vi "POP_Make Popup Visible.vi"(6 "LV Version":string, 7 "Popup Parameters":T1={"Prop Type"=enum."Unkown", "Initial Value"=variant, "Caption Strings"=[], "Ring Strings"=[], "Cell Rect"={"left"=0, "top"=0, "right"=0, "bottom"=0}, "Mouse Coords"={"x"=0, "y"=0}, "Call Data"=variant, "Ring Values"=[], "Browse Options"={"Prompt"="", "Match Pattern"="", "Mode"=enum."existing file", "Start Path"=path "", "Pattern Label"="", "Button Text"=""}, "Combo Box"={"Allow Undefined Strings"=FALSE}}, 8 "error in (no error)":errorcluster, 9 "Ctl Offsets":cluster{"Left":i32, "Top":i32}[](array[cluster]), 11 "Popup Cluster Ref":refnum<vi>) -> (0 "error out":errorcluster, 2 "event data":T4)   [LabVIEW 2016]
uses:
  Ctrls/POP_Monitor Register Data.ctl
  Ctrls/POP_Event Enum.ctl
  Ctrls/POP_Popup Call Parameters.ctl
  Ctrls/POP_Data Type.ctl
  <vilib>/Utility/miscctls.llb/LVBrowseOptionsTypeDef.ctl
  <vilib>/Utility/miscctls.llb/LVStringsAndValuesArrayTypeDef.ctl
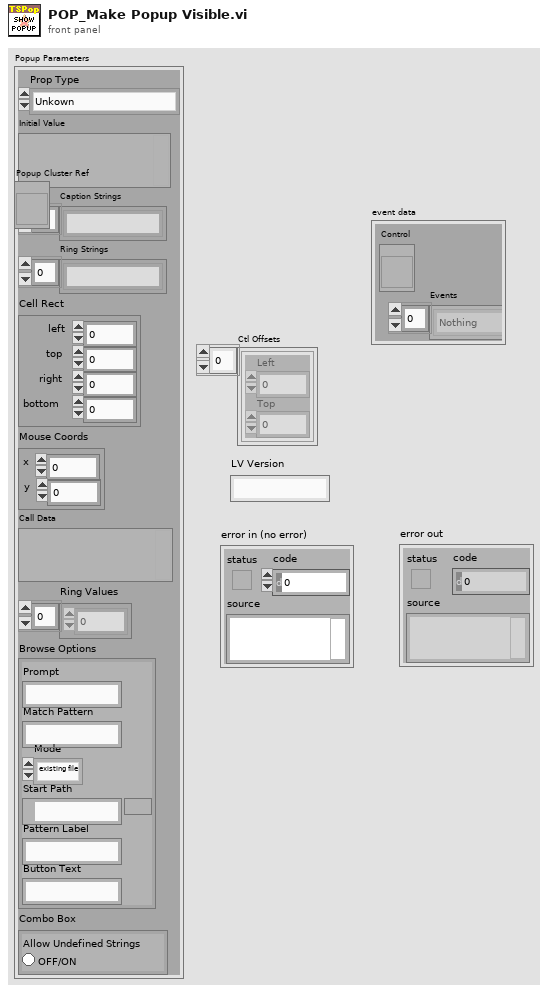
[diagram p1: front panel]
types:
  T1 = typedef "POP_Popup Call Parameters.ctl" = cluster{"Prop Type":T2, "Initial Value":variant, "Caption Strings":string[], "Ring Strings":string[], "Cell Rect":cluster{"left":i16, "top":i16, "right":i16, "bottom":i16}, "Mouse Coords":cluster{"x":i16, "y":i16}, "Call Data":variant, "Ring Values":ext[], "Browse Options":T3, "Combo Box":cluster{"Allow Undefined Strings":bool}}
  T2 = typedef "POP_Data Type.ctl" = enum16{"NO POPUP", "Unkown", "String", "Integer", "Float", "Color", "Boolean", "Ring", "Captioned String", "Captioned Integer", "Button Color", "2 Int Cluster", "4 Int Cluster", "6-Dbl Cluster", "Path", "Combox", "Time", "ShotCut String"}
  T3 = typedef "LVBrowseOptionsTypeDef.ctl" = cluster{"Prompt":string, "Match Pattern":string, "Mode":enum32{"existing file", "new file", "new or existing file", "existing dir", "new dir", "new or existing dir", "existing file (use LLBs)", "new file (use LLBs)", "new or existing file (use LLBs)", "new or existing file or directory (use LLBs)", "existing dir (use LLBs)", "new dir (use LLBs)", "new or existing dir (use LLBs)", "existing file or dir", "new file or dir", "new or existing file or dir", "existing file or dir (use LLBs)", "new file or dir (use LLBs)"}, "Start Path":path, "Pattern Label":string, "Button Text":string}
  T4 = typedef "POP_Monitor Register Data.ctl" = cluster{"Control":refnum<vi>, "Events":T5[]}
  T5 = typedef "POP_Event Enum.ctl" = enum16{"Nothing", "Enter Key Accept", "Escape Key Cancel", "Mouse Outside Accept", "Mouse Outside Cancel", "Mouse Move Accept", "Mouse Move Cancel", "Mouse Leave Cancel", "Value Change Accept", "Lose Focus Cancel", "Cancel Button", "Accept Button", "Shift Ctrl Key Down"}
  T6 = typedef "LVStringsAndValuesArrayTypeDef.ctl" = cluster{"String":string, "Value":ext}[]
  T7 = cluster{"left":i32, "top":i32, "right":i32, "bottom":i32}
  T8 = cluster{"a0":dbl, "a1":dbl, "a2":dbl, "a3":dbl, "a4":dbl, "a5":dbl}
  T9 = cluster{"left":i16, "top":i16, "right":i16, "bottom":i16}
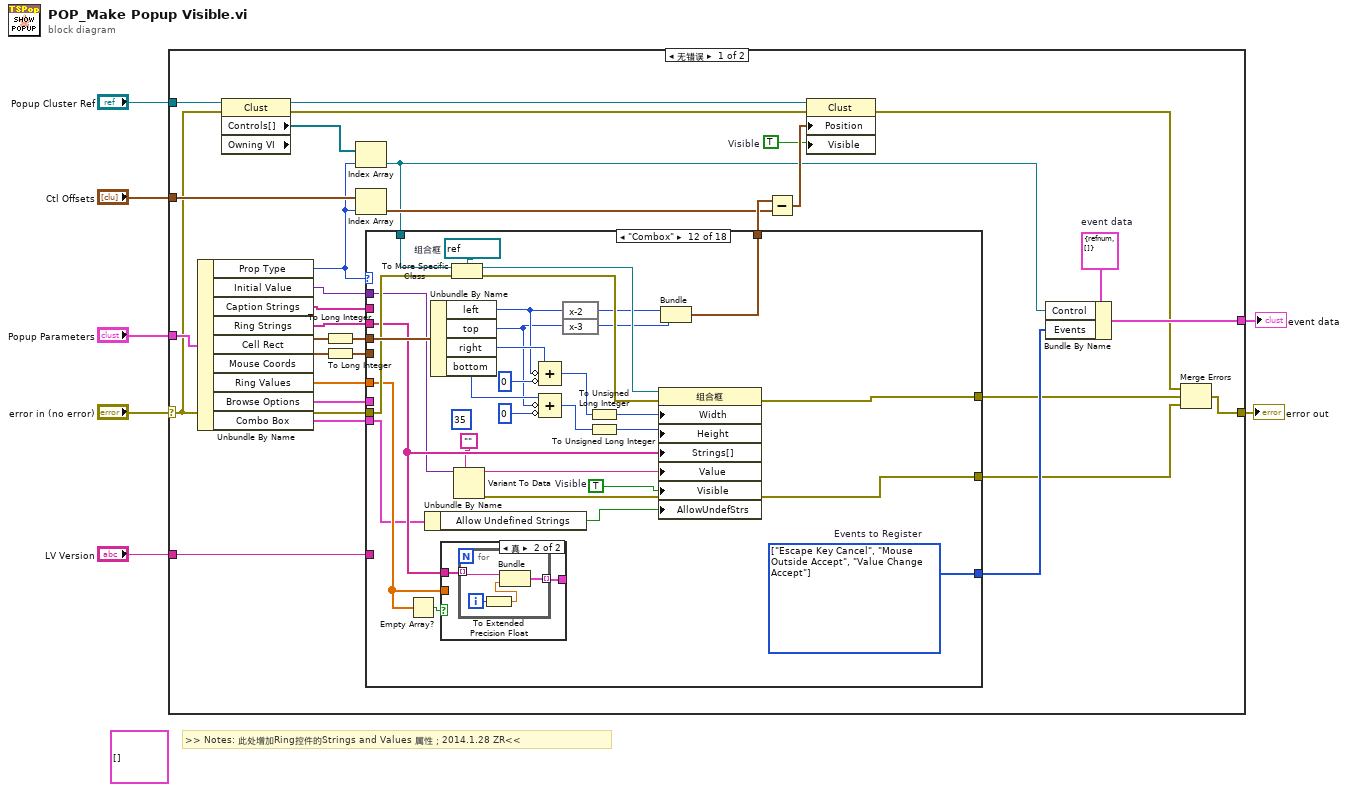
[diagram p0: block diagram]
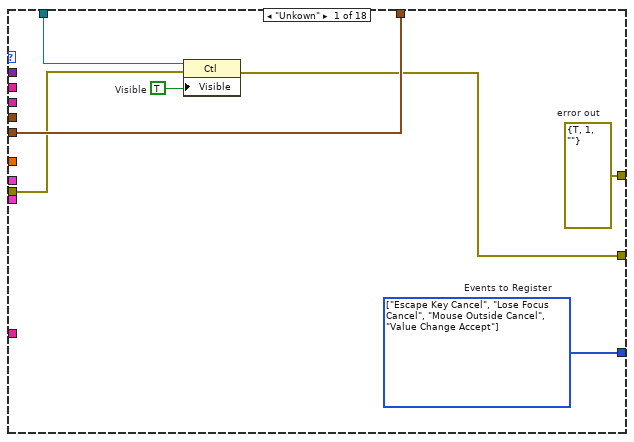
[diagram p2: hidden frame]
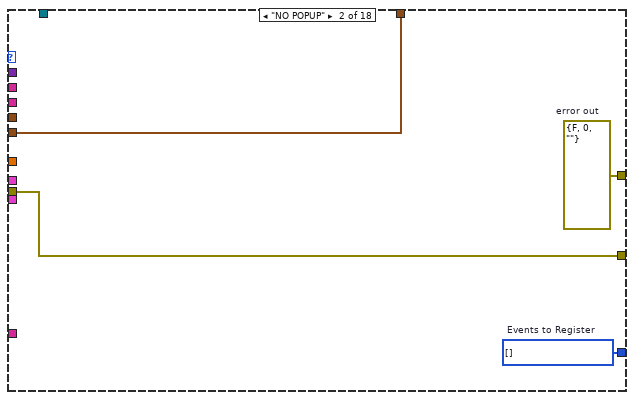
[diagram p3: hidden frame]
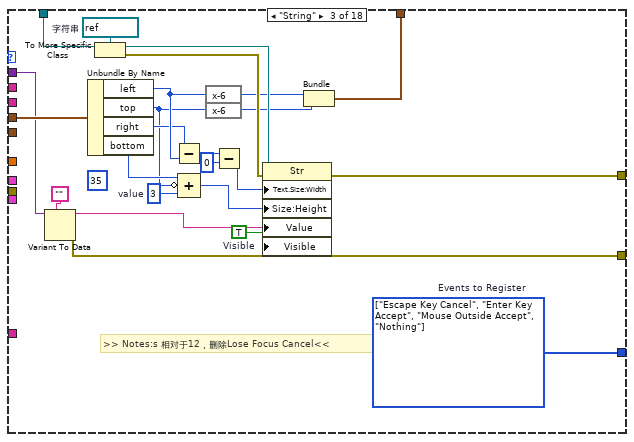
[diagram p4: hidden frame]
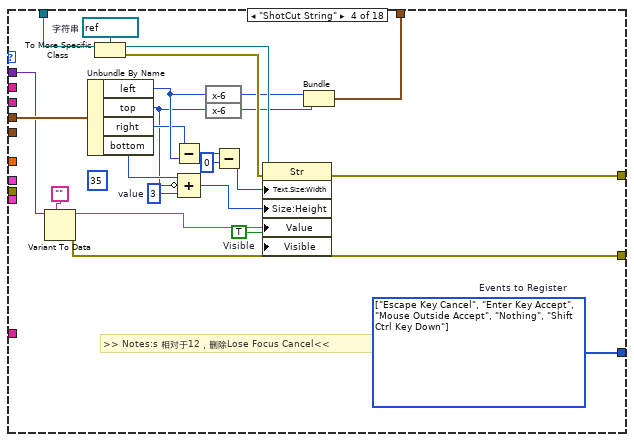
[diagram p5: hidden frame]
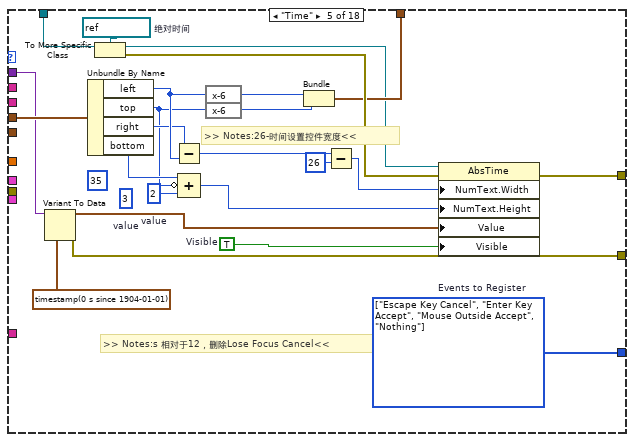
[diagram p6: hidden frame]
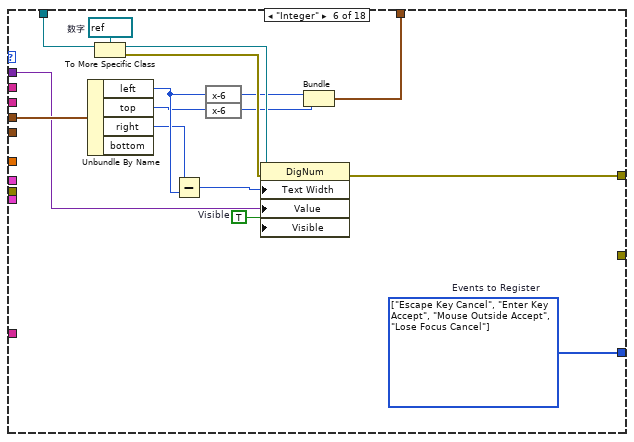
[diagram p7: hidden frame]
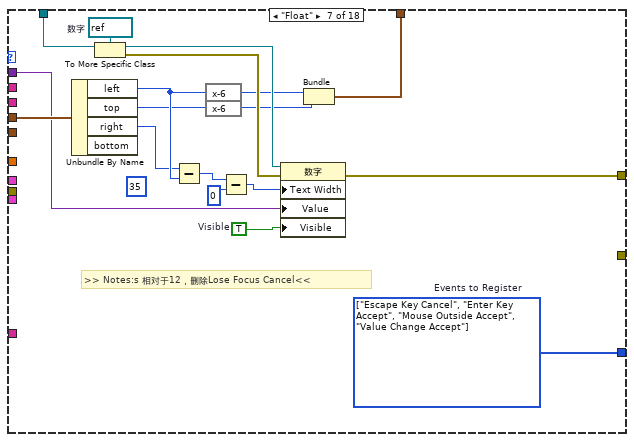
[diagram p8: hidden frame]
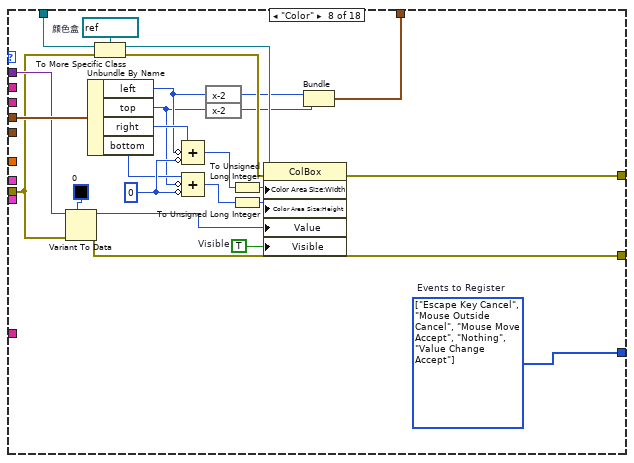
[diagram p9: hidden frame]
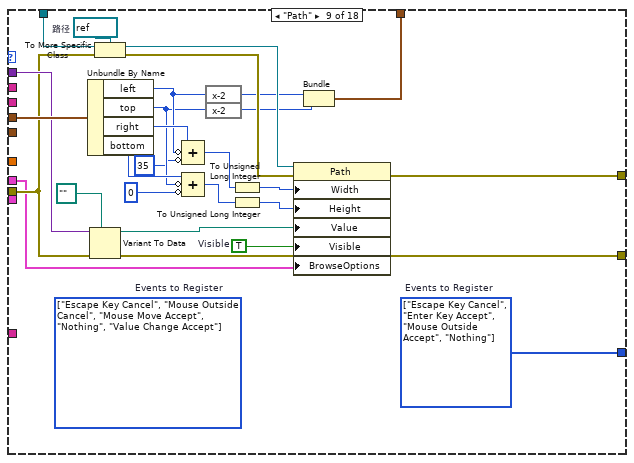
[diagram p10: hidden frame]
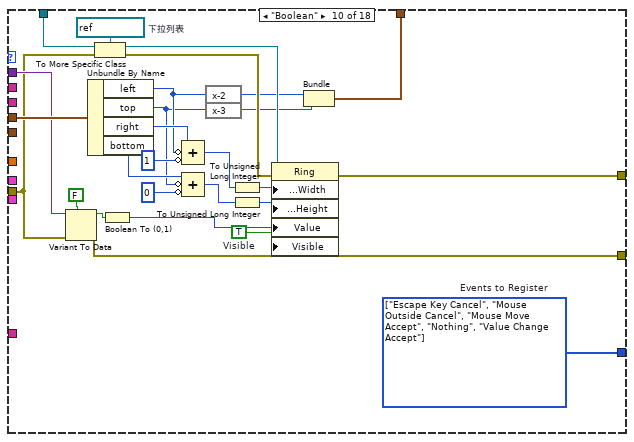
[diagram p11: hidden frame]
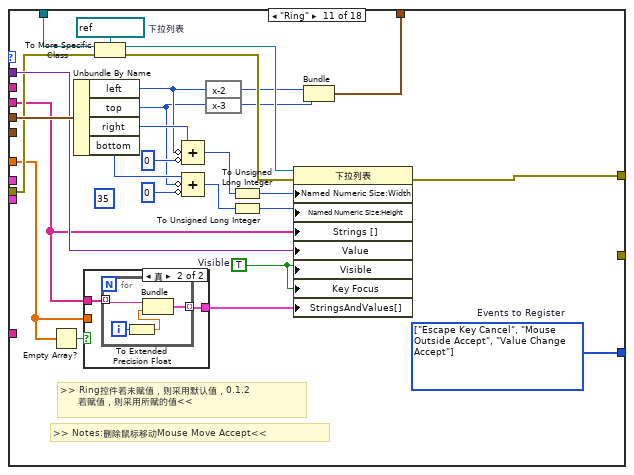
[diagram p12: hidden frame]
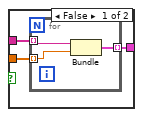
[diagram p13: hidden frame]
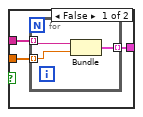
[diagram p14: hidden frame]
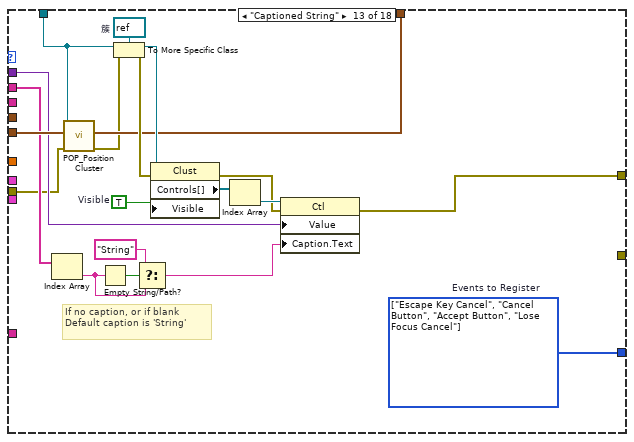
[diagram p15: hidden frame]
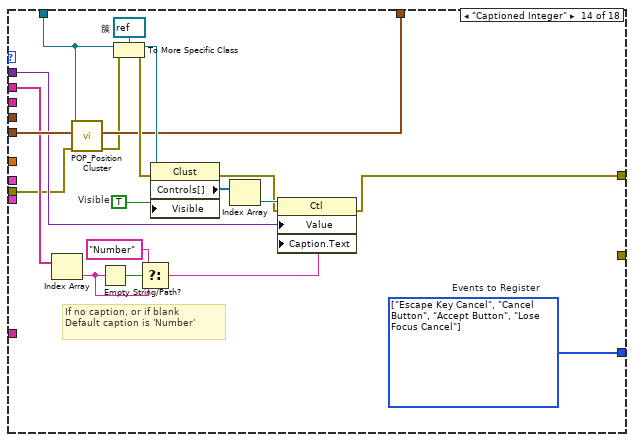
[diagram p16: hidden frame]
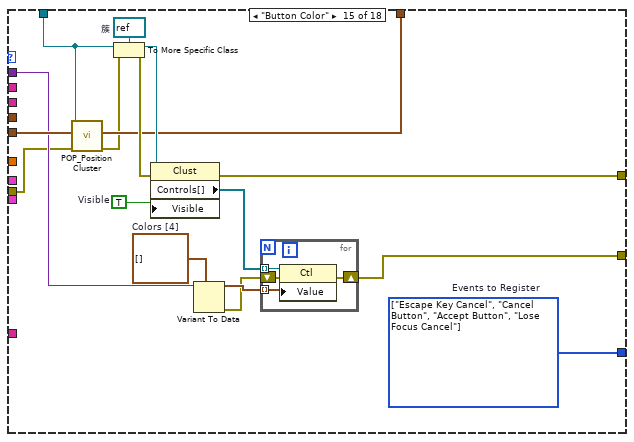
[diagram p17: hidden frame]
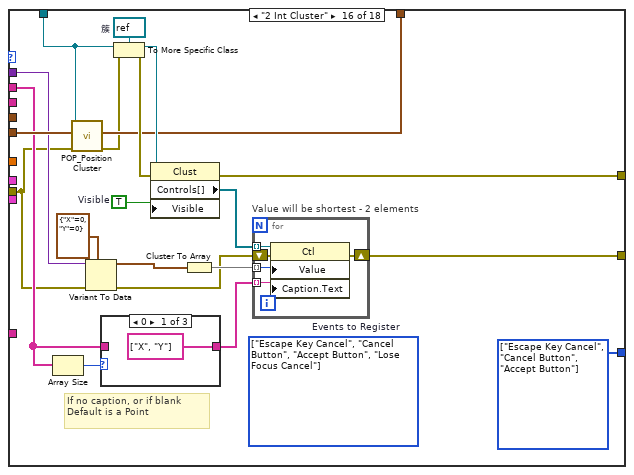
[diagram p18: hidden frame]
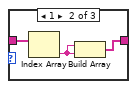
[diagram p19: hidden frame]
diagram:
  (unwired) T6 [] ("Strings And Values []")
  # ">> Notes: 此处增加Ring控件的Strings and Values 属性；2014.1.28 ZR<<"
  n1 = case shown="无错误" "error in (no error)" {
    selector: "error in (no error)" -> [w12 w490]
    tunnel: "Popup Parameters" -> [w38 _]
    tunnel: "Popup Cluster Ref" -> [w37 _]
    tunnel: "Ctl Offsets" -> [w35 _]
    tunnel: [w24 w489] -> w4
    tunnel: [w17 w490] -> w2
    tunnel: "LV Version" -> [w13 _]
    frame No Error {
      w34 = T4 {"Control"=refnum, "Events"=[]}  # event data
      w11 = TRUE  # Visible
      n2 = Unbundle By Name(w38) -> ("Prop Type"=w32:T2, "Initial Value"=w33:variant, "Caption Strings"=w22:string[], "Ring Strings"=w23:string[], "Cell Rect"=w30:T9, "Mouse Coords"=w15:cluster{"x":i16, "y":i16}, "Ring Values"=w10:ext[], "Browse Options"=w9:T3, "Combo Box"=w8:cluster{"Allow Undefined Strings":bool})
      n3 = property class="Clust" props=["Controls[]", "Owning VI"](reference=w37, error in=w12) -> (reference out=w31:refnum<vi>, error out=w21:errorcluster, "Controls[]"=w36:refnum<vi>[])  [unwired: 1 out]
      n4 = To Long Integer(number=w30) -> (32bit integer=w16:T7)
      n5 = To Long Integer(number=w15) -> (32bit integer=w14:cluster{"x":i32, "y":i32})
      n6 = Index Array(array=w36, index=w32) -> (element=w25:refnum<vi>)
      n7 = Index Array(array=w35, index=w32) -> (element=w28:cluster{"Left":i32, "Top":i32})
      n8 = case shown="\"Combox\"" w32 {
        tunnel: w25 -> [w42 _ w63 w87 w112 w133 w153 w179 w206 w232 w260 w303 w326 w346 w365 w391 w421 w461]
        tunnel: w33 -> [_ _ w66 w90 w114 w123 w143 w170 w198 w224 w242 w278 w327 w347 w362 w390 w420 w460]
        tunnel: w16 -> [_ _ w67 w91 w115 w134 w154 w180 w207 w233 w261 w304 _ _ _ _ _ _]
        tunnel: [w45 w49 w59 w83 w109 w129 w149 w175 w202 w228 w256 w299 w319 w338 w370 w395 w426 w466] -> w19
        tunnel: [w44 w47 w56 w80 w106 w126 w146 w172 w199 w225 w253 w296 w330 w350 w366 w392 w422 w462] -> w29
        tunnel: [w43 w48 w55 w79 w105 w125 w145 w158 w183 w209 w240 w284 w333 w353 w369 w378 w425 w465] -> w26
        tunnel: w23 -> [_ _ _ _ _ _ _ _ _ _ w238 w282 _ _ _ _ _ _]
        tunnel: w14 -> [w44 w47 _ _ _ _ _ _ _ _ _ _ w331 w351 w367 w393 w423 w463]
        tunnel: w22 -> [_ _ _ _ _ _ _ _ _ _ _ _ w325 w345 _ w388 w418 w458]
        tunnel: [w39 w46 w52 w76 w102 _ _ w159 w188 w210 _ w276 _ _ w358 w384 w410 w451] -> w18
        tunnel: w13 -> [_ _ _ _ _ _ _ _ _ _ _ _ _ _ _ _ _ _]
        tunnel: w12 -> [w40 w46 _ _ _ _ _ w157 w187 w208 w241 w285 w317 w337 w357 w379 w409 w450]
        tunnel: w10 -> [_ _ _ _ _ _ _ _ _ _ w236 w281 _ _ _ _ _ _]
        tunnel: w9 -> [_ _ _ _ _ _ _ _ w181 _ _ _ _ _ _ _ _ _]
        tunnel: w8 -> [_ _ _ _ _ _ _ _ _ _ _ w275 _ _ _ _ _ _]
        frame "Unkown" {
          w43 = T5[] [enum."Escape Key Cancel", enum."Lose Focus Cancel", enum."Mouse Outside Cancel", enum."Value Change Accept"] items=["Nothing", "Enter Key Accept", "Escape Key Cancel", "Mouse Outside Accept", "Mouse Outside Cancel", "Mouse Move Accept", "Mouse Move Cancel", "Mouse Leave Cancel", "Value Change Accept", "Lose Focus Cancel", "Cancel Button", "Accept Button", "Shift Ctrl Key Down"]  # Events to Register
          w45 = errorcluster {"status"=TRUE, "code"=1, "source"=""}  # error out
          w41 = TRUE  # Visible
          n9 = property class="Ctl"(reference=w42, error in=w40, "Visible"=w41) -> (error out=w39:errorcluster)  [unwired: 1 out]
        }
        frame "NO POPUP" {
          w48 = T5[] [] items=["Nothing", "Enter Key Accept", "Escape Key Cancel", "Mouse Outside Accept", "Mouse Outside Cancel", "Mouse Move Accept", "Mouse Move Cancel", "Mouse Leave Cancel", "Value Change Accept", "Lose Focus Cancel", "Cancel Button", "Accept Button", "Shift Ctrl Key Down"]  # Events to Register
          w49 = errorcluster {"status"=FALSE, "code"=0, "source"=""}  # error out
        }
        frame "String" {
          (unwired) 35 ("y")
          w62 = refnum<vi> refnum  # 字符串
          w68 = TRUE  # Visible
          w69 = 3  # value
          w55 = T5[] [enum."Escape Key Cancel", enum."Enter Key Accept", enum."Mouse Outside Accept", enum."Nothing"] items=["Nothing", "Enter Key Accept", "Escape Key Cancel", "Mouse Outside Accept", "Mouse Outside Cancel", "Mouse Move Accept", "Mouse Move Cancel", "Mouse Leave Cancel", "Value Change Accept", "Lose Focus Cancel", "Cancel Button", "Accept Button", "Shift Ctrl Key Down"]  # Events to Register
          # ">> Notes:s 相对于12，删除Lose Focus Cancel<<"
          n10 = Variant To Data(type="", Variant=w66) -> (data=w64:string, error out=w52:errorcluster)  [unwired: 1 in]
          n11 = Unbundle By Name(w67) -> ("left"=w71:i32, "top"=w53:i32, "right"=w54:i32, "bottom"=w73:i32)
          n12 = To More Specific Class(target class=w62, reference=w63) -> (specific class reference=w61:refnum<vi>, error out=w60:errorcluster)  [unwired: 1 in]
          n13 = Subtract(x=w54, y=w71) -> (x-y=w70:i32)
          n14 = Compound Arithmetic op=ADD(w73, invert w53, w69) -> (w72:i32)
          n15 = expression code="x-6"(w71) -> (w58:i32)
          n16 = expression code="x-6"(w53) -> (w57:i32)
          n17 = Subtract(x=w70, y=0) -> (x-y=w51:i32)
          n18 = property class="Str"(reference=w61, error in=w60, "Text.Size:Width"=w51, "Size:Height"=w72, "Value"=w64, "Visible"=w68) -> (error out=w59:errorcluster)  [unwired: 1 out]
          n19 = Bundle("left"=w58, "top"=w57) -> (w56:cluster{"left":i32, "top":i32})  [unwired: 1 in]
        }
        frame "ShotCut String" {
          (unwired) 35 ("y")
          w86 = refnum<vi> refnum  # 字符串
          w92 = TRUE  # Visible
          w93 = 3  # value
          w79 = T5[] [enum."Escape Key Cancel", enum."Enter Key Accept", enum."Mouse Outside Accept", enum."Nothing", enum."Shift Ctrl Key Down"] items=["Nothing", "Enter Key Accept", "Escape Key Cancel", "Mouse Outside Accept", "Mouse Outside Cancel", "Mouse Move Accept", "Mouse Move Cancel", "Mouse Leave Cancel", "Value Change Accept", "Lose Focus Cancel", "Cancel Button", "Accept Button", "Shift Ctrl Key Down"]  # Events to Register
          # ">> Notes:s 相对于12，删除Lose Focus Cancel<<"
          n20 = Variant To Data(type="", Variant=w90) -> (data=w88:string, error out=w76:errorcluster)  [unwired: 1 in]
          n21 = Unbundle By Name(w91) -> ("left"=w95:i32, "top"=w77:i32, "right"=w78:i32, "bottom"=w97:i32)
          n22 = To More Specific Class(target class=w86, reference=w87) -> (specific class reference=w85:refnum<vi>, error out=w84:errorcluster)  [unwired: 1 in]
          n23 = Subtract(x=w78, y=w95) -> (x-y=w94:i32)
          n24 = Compound Arithmetic op=ADD(w97, invert w77, w93) -> (w96:i32)
          n25 = expression code="x-6"(w95) -> (w82:i32)
          n26 = expression code="x-6"(w77) -> (w81:i32)
          n27 = Subtract(x=w94, y=0) -> (x-y=w75:i32)
          n28 = property class="Str"(reference=w85, error in=w84, "Text.Size:Width"=w75, "Size:Height"=w96, "Value"=w88, "Visible"=w92) -> (error out=w83:errorcluster)  [unwired: 1 out]
          n29 = Bundle("left"=w82, "top"=w81) -> (w80:cluster{"left":i32, "top":i32})  [unwired: 1 in]
        }
        frame "Time" {
          (unwired) 3  # value
          (unwired) 35 ("y")
          w111 = refnum<vi> refnum  # 绝对时间
          w116 = TRUE  # Visible
          w117 = 2  # value
          w105 = T5[] [enum."Escape Key Cancel", enum."Enter Key Accept", enum."Mouse Outside Accept", enum."Nothing"] items=["Nothing", "Enter Key Accept", "Escape Key Cancel", "Mouse Outside Accept", "Mouse Outside Cancel", "Mouse Move Accept", "Mouse Move Cancel", "Mouse Leave Cancel", "Value Change Accept", "Lose Focus Cancel", "Cancel Button", "Accept Button", "Shift Ctrl Key Down"]  # Events to Register
          # ">> Notes:26-时间设置控件宽度<<"
          # ">> Notes:s 相对于12，删除Lose Focus Cancel<<"
          n30 = Variant To Data(type=timestamp(0 s since 1904-01-01) ("Time"), Variant=w114) -> (data=w113:timestamp, error out=w102:errorcluster)  [unwired: 1 in]
          n31 = Unbundle By Name(w115) -> ("left"=w119:i32, "top"=w103:i32, "right"=w104:i32, "bottom"=w121:i32)
          n32 = To More Specific Class(target class=w111, reference=w112) -> (specific class reference=w98:refnum<vi>, error out=w110:errorcluster)  [unwired: 1 in]
          n33 = Subtract(x=w104, y=w119) -> (x-y=w118:i32)
          n34 = Compound Arithmetic op=ADD(w121, invert w103, w117) -> (w120:i32)
          n35 = expression code="x-6"(w119) -> (w108:i32)
          n36 = expression code="x-6"(w103) -> (w107:i32)
          n37 = Bundle("left"=w108, "top"=w107) -> (w106:cluster{"left":i32, "top":i32})  [unwired: 1 in]
          n38 = Subtract(x=w118, y=26) -> (x-y=w101:i32)
          n39 = property class="AbsTime"(reference=w98, error in=w110, "NumText.Width"=w101, "NumText.Height"=w120, "Value"=w113, "Visible"=w116) -> (error out=w109:errorcluster)  [unwired: 1 out]
        }
        frame "Integer" {
          w132 = refnum<vi> refnum  # 数字
          w135 = TRUE  # Visible
          w125 = T5[] [enum."Escape Key Cancel", enum."Enter Key Accept", enum."Mouse Outside Accept", enum."Lose Focus Cancel"] items=["Nothing", "Enter Key Accept", "Escape Key Cancel", "Mouse Outside Accept", "Mouse Outside Cancel", "Mouse Move Accept", "Mouse Move Cancel", "Mouse Leave Cancel", "Value Change Accept", "Lose Focus Cancel", "Cancel Button", "Accept Button", "Shift Ctrl Key Down"]  # Events to Register
          n40 = Unbundle By Name(w134) -> ("left"=w137:i32, "top"=w122:i32, "right"=w124:i32)  [unwired: 1 out]
          n41 = To More Specific Class(target class=w132, reference=w133) -> (specific class reference=w131:refnum<vi>, error out=w130:errorcluster)  [unwired: 1 in]
          n42 = Subtract(x=w124, y=w137) -> (x-y=w136:i32)
          n43 = expression code="x-6"(w137) -> (w128:i32)
          n44 = expression code="x-6"(w122) -> (w127:i32)
          n45 = property class="DigNum"(reference=w131, error in=w130, "Text Width"=w136, "Value"=w123, "Visible"=w135) -> (error out=w129:errorcluster)  [unwired: 1 out]
          n46 = Bundle("left"=w128, "top"=w127) -> (w126:cluster{"left":i32, "top":i32})  [unwired: 1 in]
        }
        frame "Float" {
          (unwired) 35 ("y")
          w152 = refnum<vi> refnum  # 数字
          w138 = TRUE  # Visible
          w145 = T5[] [enum."Escape Key Cancel", enum."Enter Key Accept", enum."Mouse Outside Accept", enum."Value Change Accept"] items=["Nothing", "Enter Key Accept", "Escape Key Cancel", "Mouse Outside Accept", "Mouse Outside Cancel", "Mouse Move Accept", "Mouse Move Cancel", "Mouse Leave Cancel", "Value Change Accept", "Lose Focus Cancel", "Cancel Button", "Accept Button", "Shift Ctrl Key Down"]  # Events to Register
          # ">> Notes:s 相对于12，删除Lose Focus Cancel<<"
          n47 = Unbundle By Name(w154) -> ("left"=w155:i32, "top"=w142:i32, "right"=w144:i32)  [unwired: 1 out]
          n48 = To More Specific Class(target class=w152, reference=w153) -> (specific class reference=w151:refnum<vi>, error out=w150:errorcluster)  [unwired: 1 in]
          n49 = Subtract(x=w144, y=w155) -> (x-y=w140:i32)
          n50 = expression code="x-6"(w155) -> (w148:i32)
          n51 = expression code="x-6"(w142) -> (w147:i32)
          n52 = Subtract(x=w140, y=0) -> (x-y=w139:i32)
          n53 = property class="数字"(reference=w151, error in=w150, "Text Width"=w139, "Value"=w143, "Visible"=w138) -> (error out=w149:errorcluster)  [unwired: 1 out]
          n54 = Bundle("left"=w148, "top"=w147) -> (w146:cluster{"left":i32, "top":i32})  [unwired: 1 in]
        }
        frame "Color" {
          w158 = T5[] [enum."Escape Key Cancel", enum."Mouse Outside Cancel", enum."Mouse Move Accept", enum."Nothing", enum."Value Change Accept"] items=["Nothing", "Enter Key Accept", "Escape Key Cancel", "Mouse Outside Accept", "Mouse Outside Cancel", "Mouse Move Accept", "Mouse Move Cancel", "Mouse Leave Cancel", "Value Change Accept", "Lose Focus Cancel", "Cancel Button", "Accept Button", "Shift Ctrl Key Down"]  # Events to Register
          w178 = refnum<vi> refnum  # 颜色盒
          w168 = 0
          w156 = TRUE  # Visible
          n55 = Variant To Data(error in=w157, type=u32 0, Variant=w170) -> (data=w169:u32, error out=w159:errorcluster)
          n56 = Unbundle By Name(w180) -> ("left"=w166:i32, "top"=w164:i32, "right"=w167:i32, "bottom"=w165:i32)
          n57 = To More Specific Class(target class=w178, reference=w179, error in=w157) -> (specific class reference=w177:refnum<vi>, error out=w176:errorcluster)
          n58 = Compound Arithmetic op=ADD(w167, invert w166, invert w168) -> (w162:i32)
          n59 = Compound Arithmetic op=ADD(w165, invert w164, invert w168) -> (w163:i32)
          n60 = expression code="x-2"(w166) -> (w174:i32)
          n61 = expression code="x-2"(w164) -> (w173:i32)
          n62 = To Unsigned Long Integer(number=w162) -> (unsigned 32bit integer=w161:u32)
          n63 = To Unsigned Long Integer(number=w163) -> (unsigned 32bit integer=w160:u32)
          n64 = property class="ColBox"(reference=w177, error in=w176, "Color Area Size:Width"=w161, "Color Area Size:Height"=w160, "Value"=w169, "Visible"=w156) -> (error out=w175:errorcluster)  [unwired: 1 out]
          n65 = Bundle("left"=w174, "top"=w173) -> (w172:cluster{"left":i32, "top":i32})  [unwired: 1 in]
        }
        frame "Path" {
          w183 = T5[] [enum."Escape Key Cancel", enum."Enter Key Accept", enum."Mouse Outside Accept", enum."Nothing"] items=["Nothing", "Enter Key Accept", "Escape Key Cancel", "Mouse Outside Accept", "Mouse Outside Cancel", "Mouse Move Accept", "Mouse Move Cancel", "Mouse Leave Cancel", "Value Change Accept", "Lose Focus Cancel", "Cancel Button", "Accept Button", "Shift Ctrl Key Down"]  # Events to Register
          (unwired) T5[] [enum."Escape Key Cancel", enum."Mouse Outside Cancel", enum."Mouse Move Accept", enum."Nothing", enum."Value Change Accept"] items=["Nothing", "Enter Key Accept", "Escape Key Cancel", "Mouse Outside Accept", "Mouse Outside Cancel", "Mouse Move Accept", "Mouse Move Cancel", "Mouse Leave Cancel", "Value Change Accept", "Lose Focus Cancel", "Cancel Button", "Accept Button", "Shift Ctrl Key Down"]  # Events to Register
          w205 = refnum<vi> refnum  # 路径
          w186 = TRUE  # Visible
          n66 = Unbundle By Name(w207) -> ("left"=w195:i32, "top"=w193:i32, "right"=w196:i32, "bottom"=w194:i32)
          n67 = Variant To Data(error in=w187, type=path "" ("值"), Variant=w198) -> (data=w184:path, error out=w188:errorcluster)
          n68 = To More Specific Class(target class=w205, reference=w206, error in=w187) -> (specific class reference=w204:refnum<vi>, error out=w203:errorcluster)
          n69 = Compound Arithmetic op=ADD(w196, invert w195, invert 35 ("值")) -> (w191:i32)
          n70 = Compound Arithmetic op=ADD(w194, invert w193, invert 0) -> (w192:i32)
          n71 = expression code="x-2"(w195) -> (w201:i32)
          n72 = expression code="x-2"(w193) -> (w200:i32)
          n73 = To Unsigned Long Integer(number=w191) -> (unsigned 32bit integer=w190:u32)
          n74 = To Unsigned Long Integer(number=w192) -> (unsigned 32bit integer=w189:u32)
          n75 = property class="Path"(reference=w204, error in=w203, "Width"=w190, "Height"=w189, "Value"=w184, "Visible"=w186, "BrowseOptions"=w181) -> (error out=w202:errorcluster)  [unwired: 1 out]
          n76 = Bundle("left"=w201, "top"=w200) -> (w199:cluster{"left":i32, "top":i32})  [unwired: 1 in]
        }
        frame "Boolean" {
          w209 = T5[] [enum."Escape Key Cancel", enum."Mouse Outside Cancel", enum."Mouse Move Accept", enum."Nothing", enum."Value Change Accept"] items=["Nothing", "Enter Key Accept", "Escape Key Cancel", "Mouse Outside Accept", "Mouse Outside Cancel", "Mouse Move Accept", "Mouse Move Cancel", "Mouse Leave Cancel", "Value Change Accept", "Lose Focus Cancel", "Cancel Button", "Accept Button", "Shift Ctrl Key Down"]  # Events to Register
          w231 = refnum<vi> refnum  # 下拉列表
          w234 = TRUE  # Visible
          n77 = Variant To Data(error in=w208, type=FALSE, Variant=w224) -> (data=w223:bool, error out=w210:errorcluster)
          n78 = Unbundle By Name(w233) -> ("left"=w220:i32, "top"=w218:i32, "right"=w221:i32, "bottom"=w219:i32)
          n79 = To More Specific Class(target class=w231, reference=w232, error in=w208) -> (specific class reference=w230:refnum<vi>, error out=w229:errorcluster)
          n80 = Boolean To (0,1)(Boolean=w223) -> (0, 1=w212:i16)
          n81 = Compound Arithmetic op=ADD(w221, invert w220, invert 1) -> (w216:i32)
          n82 = Compound Arithmetic op=ADD(w219, invert w218, invert 0) -> (w217:i32)
          n83 = expression code="x-2"(w220) -> (w227:i32)
          n84 = expression code="x-3"(w218) -> (w226:i32)
          n85 = To Unsigned Long Integer(number=w216) -> (unsigned 32bit integer=w215:u32)
          n86 = To Unsigned Long Integer(number=w217) -> (unsigned 32bit integer=w214:u32)
          n87 = property class="Ring"(reference=w230, error in=w229, "Named Numeric Size:Width"=w215, "Named Numeric Size:Height"=w214, "Value"=w212, "Visible"=w234) -> (error out=w228:errorcluster)  [unwired: 1 out]
          n88 = Bundle("left"=w227, "top"=w226) -> (w225:cluster{"left":i32, "top":i32})  [unwired: 1 in]
        }
        frame "Ring" {
          (unwired) 35
          w240 = T5[] [enum."Escape Key Cancel", enum."Mouse Outside Accept", enum."Value Change Accept"] items=["Nothing", "Enter Key Accept", "Escape Key Cancel", "Mouse Outside Accept", "Mouse Outside Cancel", "Mouse Move Accept", "Mouse Move Cancel", "Mouse Leave Cancel", "Value Change Accept", "Lose Focus Cancel", "Cancel Button", "Accept Button", "Shift Ctrl Key Down"]  # Events to Register
          w259 = refnum<vi> refnum  # 下拉列表
          w239 = TRUE  # Visible
          # ">> Ring控件若未赋值，则采用默认值，0.1.2\n      若赋值，则采用所赋的值<<"
          # ">> Notes:删除鼠标移动Mouse Move Accept<<"
          n89 = Empty Array?(array=w236) -> (empty?=w235:bool)
          n90 = Unbundle By Name(w261) -> ("left"=w250:i32, "top"=w248:i32, "right"=w251:i32, "bottom"=w249:i32)
          n91 = case shown="真" w235 {
            tunnel: w238 -> [w264 w269]
            tunnel: [w263 w268] -> w237
            tunnel: w236 -> [w262 _]
            frame False {
              n92 = for {
                tunnel: w264 -> [w267] mode=indexing
                tunnel: w262 -> [w266] mode=indexing
                tunnel: [w265] -> w263 mode=indexing
                n93 = Bundle("String"=w267, "Value"=w266) -> (w265:cluster{"String":string, "Value":ext})  [unwired: 1 in]
              }
            }
            frame True {
              n94 = for {
                tunnel: w269 -> [w273] mode=indexing
                tunnel: [w272] -> w268 mode=indexing
                i -> [w270]
                n95 = To Extended Precision Float(1:w270) -> (0:w271:ext)
                n96 = Bundle("String"=w273, w271) -> (w272:cluster{"String":string, ext})  [unwired: 1 in]
              }
            }
          }
          n97 = To More Specific Class(target class=w259, reference=w260, error in=w241) -> (specific class reference=w258:refnum<vi>, error out=w257:errorcluster)
          n98 = Compound Arithmetic op=ADD(w251, invert w250, invert 0) -> (w246:i32)
          n99 = Compound Arithmetic op=ADD(w249, invert w248, invert 0) -> (w247:i32)
          n100 = expression code="x-2"(w250) -> (w255:i32)
          n101 = expression code="x-3"(w248) -> (w254:i32)
          n102 = To Unsigned Long Integer(number=w246) -> (unsigned 32bit integer=w245:u32)
          n103 = To Unsigned Long Integer(number=w247) -> (unsigned 32bit integer=w244:u32)
          n104 = property class="下拉列表"(reference=w258, error in=w257, "Named Numeric Size:Width"=w245, "Named Numeric Size:Height"=w244, "Strings []"=w238, "Value"=w242, "Visible"=w239, "Key Focus"=w239, "StringsAndValues[]"=w237) -> (error out=w256:errorcluster)  [unwired: 1 out]
          n105 = Bundle("left"=w255, "top"=w254) -> (w253:cluster{"left":i32, "top":i32})  [unwired: 1 in]
        }
        frame "Combox" {
          (unwired) 35
          w284 = T5[] [enum."Escape Key Cancel", enum."Mouse Outside Accept", enum."Value Change Accept"] items=["Nothing", "Enter Key Accept", "Escape Key Cancel", "Mouse Outside Accept", "Mouse Outside Cancel", "Mouse Move Accept", "Mouse Move Cancel", "Mouse Leave Cancel", "Value Change Accept", "Lose Focus Cancel", "Cancel Button", "Accept Button", "Shift Ctrl Key Down"]  # Events to Register
          w302 = refnum<vi> refnum  # 组合框
          w283 = TRUE  # Visible
          n106 = Empty Array?(array=w281) -> (empty?=w280:bool)
          n107 = Unbundle By Name(w275) -> ("Allow Undefined Strings"=w274:bool)
          n108 = Unbundle By Name(w304) -> ("left"=w293:i32, "top"=w291:i32, "right"=w294:i32, "bottom"=w292:i32)
          n109 = case shown="真" w280 {
            tunnel: w282 -> [w307 w312]
            tunnel: [w306 w311] -> _
            tunnel: w281 -> [w305 _]
            frame False {
              n110 = for {
                tunnel: w307 -> [w310] mode=indexing
                tunnel: w305 -> [w309] mode=indexing
                tunnel: [w308] -> w306 mode=indexing
                n111 = Bundle("String"=w310, "Value"=w309) -> (w308:cluster{"String":string, "Value":ext})  [unwired: 1 in]
              }
            }
            frame True {
              n112 = for {
                tunnel: w312 -> [w316] mode=indexing
                tunnel: [w315] -> w311 mode=indexing
                i -> [w313]
                n113 = To Extended Precision Float(1:w313) -> (0:w314:ext)
                n114 = Bundle("String"=w316, w314) -> (w315:cluster{"String":string, ext})  [unwired: 1 in]
              }
            }
          }
          n115 = To More Specific Class(target class=w302, reference=w303, error in=w285) -> (specific class reference=w301:refnum<vi>, error out=w300:errorcluster)
          n116 = Variant To Data(type="", Variant=w278) -> (data=w277:string, error out=w276:errorcluster)  [unwired: 1 in]
          n117 = Compound Arithmetic op=ADD(w294, invert w293, invert 0) -> (w289:i32)
          n118 = Compound Arithmetic op=ADD(w292, invert w291, invert 0) -> (w290:i32)
          n119 = expression code="x-2"(w293) -> (w298:i32)
          n120 = expression code="x-3"(w291) -> (w297:i32)
          n121 = To Unsigned Long Integer(number=w289) -> (unsigned 32bit integer=w288:u32)
          n122 = To Unsigned Long Integer(number=w290) -> (unsigned 32bit integer=w287:u32)
          n123 = property class="组合框"(reference=w301, error in=w300, "Width"=w288, "Height"=w287, "Strings[]"=w282, "Value"=w277, "Visible"=w283, "AllowUndefStrs"=w274) -> (error out=w299:errorcluster)  [unwired: 1 out]
          n124 = Bundle("left"=w298, "top"=w297) -> (w296:cluster{"left":i32, "top":i32})  [unwired: 1 in]
        }
        frame "Captioned String" {
          w336 = refnum<vi> refnum  # 簇
          w332 = TRUE  # Visible
          w333 = T5[] [enum."Escape Key Cancel", enum."Cancel Button", enum."Accept Button", enum."Lose Focus Cancel"] items=["Nothing", "Enter Key Accept", "Escape Key Cancel", "Mouse Outside Accept", "Mouse Outside Cancel", "Mouse Move Accept", "Mouse Move Cancel", "Mouse Leave Cancel", "Value Change Accept", "Lose Focus Cancel", "Cancel Button", "Accept Button", "Shift Ctrl Key Down"]  # Events to Register
          # "If no caption, or if blank\nDefault caption is 'String'"
          n125 = Index Array(array=w325) -> (element=w323:string)  [unwired: 1 in]
          n126 = call "POP_Position Cluster.vi"("error in (no error)"=w317, "Mouse Coords"=w331, "Ctl Refnum"=w326) -> ("error out"=w318:errorcluster, "Cluster Pos"=w330:cluster{"x":i32, "y":i32})  [unwired: 6 in, 1 out]
          n127 = Empty String/Path?(string/path=w323) -> (empty?=w324:bool)
          n128 = To More Specific Class(target class=w336, reference=w326, error in=w318) -> (specific class reference=w335:refnum<vi>, error out=w334:errorcluster)
          n129 = Select(t="String", s=w324, f=w323) -> (s? t:f=w321:string)
          n130 = property class="Clust"(reference=w335, error in=w334, "Visible"=w332) -> (error out=w320:errorcluster, "Controls[]"=w328:refnum<vi>[])  [unwired: 1 out]
          n131 = Index Array(array=w328) -> (element=w329:refnum<vi>)  [unwired: 1 in]
          n132 = property class="Ctl"(reference=w329, error in=w320, "Value"=w327, "Caption.Text"=w321) -> (error out=w319:errorcluster)  [unwired: 1 out]
        }
        frame "Captioned Integer" {
          w356 = refnum<vi> refnum  # 簇
          w352 = TRUE  # Visible
          w353 = T5[] [enum."Escape Key Cancel", enum."Cancel Button", enum."Accept Button", enum."Lose Focus Cancel"] items=["Nothing", "Enter Key Accept", "Escape Key Cancel", "Mouse Outside Accept", "Mouse Outside Cancel", "Mouse Move Accept", "Mouse Move Cancel", "Mouse Leave Cancel", "Value Change Accept", "Lose Focus Cancel", "Cancel Button", "Accept Button", "Shift Ctrl Key Down"]  # Events to Register
          # "If no caption, or if blank\nDefault caption is 'Number'"
          n133 = Index Array(array=w345) -> (element=w343:string)  [unwired: 1 in]
          n134 = call "POP_Position Cluster.vi"("error in (no error)"=w337, "Mouse Coords"=w351, "Ctl Refnum"=w346) -> ("error out"=w340:errorcluster, "Cluster Pos"=w350:cluster{"x":i32, "y":i32})  [unwired: 6 in, 1 out]
          n135 = Empty String/Path?(string/path=w343) -> (empty?=w344:bool)
          n136 = To More Specific Class(target class=w356, reference=w346, error in=w340) -> (specific class reference=w355:refnum<vi>, error out=w354:errorcluster)
          n137 = Select(t="Number", s=w344, f=w343) -> (s? t:f=w341:string)
          n138 = property class="Clust"(reference=w355, error in=w354, "Visible"=w352) -> (error out=w339:errorcluster, "Controls[]"=w348:refnum<vi>[])  [unwired: 1 out]
          n139 = Index Array(array=w348) -> (element=w349:refnum<vi>)  [unwired: 1 in]
          n140 = property class="Ctl"(reference=w349, error in=w339, "Value"=w347, "Caption.Text"=w341) -> (error out=w338:errorcluster)  [unwired: 1 out]
        }
        frame "Button Color" {
          w364 = cluster{u32, u32}[] []  # Colors [4]
          w373 = refnum<vi> refnum  # 簇
          w368 = TRUE  # Visible
          w369 = T5[] [enum."Escape Key Cancel", enum."Cancel Button", enum."Accept Button", enum."Lose Focus Cancel"] items=["Nothing", "Enter Key Accept", "Escape Key Cancel", "Mouse Outside Accept", "Mouse Outside Cancel", "Mouse Move Accept", "Mouse Move Cancel", "Mouse Leave Cancel", "Value Change Accept", "Lose Focus Cancel", "Cancel Button", "Accept Button", "Shift Ctrl Key Down"]  # Events to Register
          n141 = call "POP_Position Cluster.vi"("error in (no error)"=w357, "Mouse Coords"=w367, "Ctl Refnum"=w365) -> ("error out"=w360:errorcluster, "Cluster Pos"=w366:cluster{"x":i32, "y":i32})  [unwired: 6 in, 1 out]
          n142 = To More Specific Class(target class=w373, reference=w365, error in=w360) -> (specific class reference=w372:refnum<vi>, error out=w371:errorcluster)
          n143 = property class="Clust"(reference=w372, error in=w371, "Visible"=w368) -> (error out=w370:errorcluster, "Controls[]"=w361:refnum<vi>[])  [unwired: 1 out]
          n144 = Variant To Data(type=w364, Variant=w362) -> (data=w363:cluster{u32, u32}[], error out=w359:errorcluster)  [unwired: 1 in]
          n145 = for {
            tunnel: w363 -> [w376] mode=indexing
            tunnel: w361 -> [w377] mode=indexing
            shift-right: [w374] -> w358
            shift-left: w359 -> [w375]
            n146 = property class="Ctl"(reference=w377, error in=w375, "Value"=w376) -> (error out=w374:errorcluster)  [unwired: 1 out]
          }
        }
        frame "2 Int Cluster" {
          w378 = T5[] [enum."Escape Key Cancel", enum."Cancel Button", enum."Accept Button"] items=["Nothing", "Enter Key Accept", "Escape Key Cancel", "Mouse Outside Accept", "Mouse Outside Cancel", "Mouse Move Accept", "Mouse Move Cancel", "Mouse Leave Cancel", "Value Change Accept", "Lose Focus Cancel", "Cancel Button", "Accept Button", "Shift Ctrl Key Down"] ("Events to Register")
          w398 = refnum<vi> refnum  # 簇
          w394 = TRUE  # Visible
          (unwired) T5[] [enum."Escape Key Cancel", enum."Cancel Button", enum."Accept Button", enum."Lose Focus Cancel"] items=["Nothing", "Enter Key Accept", "Escape Key Cancel", "Mouse Outside Accept", "Mouse Outside Cancel", "Mouse Move Accept", "Mouse Move Cancel", "Mouse Leave Cancel", "Value Change Accept", "Lose Focus Cancel", "Cancel Button", "Accept Button", "Shift Ctrl Key Down"]  # Events to Register
          # "If no caption, or if blank\nDefault is a Point"
          n147 = Array Size(array=w388) -> (size(s)=w389:i32)
          n148 = call "POP_Position Cluster.vi"("error in (no error)"=w379, "Mouse Coords"=w393, "Ctl Refnum"=w391) -> ("error out"=w385:errorcluster, "Cluster Pos"=w392:cluster{"x":i32, "y":i32})  [unwired: 6 in, 1 out]
          n149 = Variant To Data(error in=w379, type=cluster{"X":i32, "Y":i32} {"X"=0, "Y"=0}, Variant=w390) -> (data=w380:cluster{"X":i32, "Y":i32}, error out=w381:errorcluster)
          n150 = case shown="0" w389 {
            tunnel: w388 -> [_ w407 w408]
            tunnel: [string[] ["X", "Y"] w405 w408] -> w387
            frame 0 {
            }
            frame 1 {
              n151 = Index Array(array=w407) -> (element=w406:string)  [unwired: 1 in]
              n152 = Build Array(w406, w406) -> (w405:string[])
            }
            frame 2, Default {
            }
          }
          n153 = To More Specific Class(target class=w398, reference=w391, error in=w385) -> (specific class reference=w397:refnum<vi>, error out=w396:errorcluster)
          n154 = property class="Clust"(reference=w397, error in=w396, "Visible"=w394) -> (error out=w395:errorcluster, "Controls[]"=w386:refnum<vi>[])  [unwired: 1 out]
          n155 = Cluster To Array(cluster=w380) -> (array=w382:i32[])
          n156 = for "Value will be shortest - 2 elements" {
            tunnel: w382 -> [w403] mode=indexing
            tunnel: w387 -> [w402] mode=indexing
            tunnel: w386 -> [w401] mode=indexing
            shift-right: [w399] -> w384
            shift-left: w381 -> [w400]
            n157 = property class="Ctl"(reference=w401, error in=w400, "Value"=w403, "Caption.Text"=w402) -> (error out=w399:errorcluster)  [unwired: 1 out]
          }
        }
        frame "4 Int Cluster" {
          w429 = refnum<vi> refnum  # 簇
          w424 = TRUE  # Visible
          w425 = T5[] [enum."Escape Key Cancel", enum."Cancel Button", enum."Accept Button", enum."Lose Focus Cancel"] items=["Nothing", "Enter Key Accept", "Escape Key Cancel", "Mouse Outside Accept", "Mouse Outside Cancel", "Mouse Move Accept", "Mouse Move Cancel", "Mouse Leave Cancel", "Value Change Accept", "Lose Focus Cancel", "Cancel Button", "Accept Button", "Shift Ctrl Key Down"]  # Events to Register
          # "If no caption, or if blank\nDefault is a Rect"
          n158 = Array Size(array=w418) -> (size(s)=w419:i32)
          n159 = call "POP_Position Cluster.vi"("error in (no error)"=w409, "Mouse Coords"=w423, "Ctl Refnum"=w421) -> ("error out"=w412:errorcluster, "Cluster Pos"=w422:cluster{"x":i32, "y":i32})  [unwired: 6 in, 1 out]
          n160 = Variant To Data(error in=w409, type=T7 {"left"=0, "top"=0, "right"=0, "bottom"=0} ("rect"), Variant=w420) -> (data=w415:T7, error out=w411:errorcluster)
          n161 = case shown="2" w419 {
            tunnel: w418 -> [_ w438 w442 w447 w448]
            tunnel: [string[] ["Left", "Top", "Right", "Bottom"] w437 w441 w446 w448] -> w417
            frame 0 {
            }
            frame 1 {
              n162 = Index Array(array=w438) -> (element=w436:string)  [unwired: 1 in]
              n163 = Build Array(w436, w436, w436, w436) -> (w437:string[])
            }
            frame 2 {
              n164 = Index Array(array=w442) -> (element #1=w440:string, element #2=w439:string)  [unwired: 2 in]
              n165 = Build Array(w440, w439, w439, w439) -> (w441:string[])
            }
            frame 3 {
              n166 = Index Array(array=w447) -> (element #1=w445:string, element #2=w444:string, element #3=w443:string)  [unwired: 3 in]
              n167 = Build Array(w445, w444, w443, w443) -> (w446:string[])
            }
            frame 4, Default {
            }
          }
          n168 = To More Specific Class(target class=w429, reference=w421, error in=w412) -> (specific class reference=w428:refnum<vi>, error out=w427:errorcluster)
          n169 = Cluster To Array(cluster=w415) -> (array=w414:i32[])
          n170 = property class="Clust"(reference=w428, error in=w427, "Visible"=w424) -> (error out=w426:errorcluster, "Controls[]"=w416:refnum<vi>[])  [unwired: 1 out]
          n171 = for "Value will be shortest - 4 elements" {
            tunnel: w414 -> [w434] mode=indexing
            tunnel: w417 -> [w433] mode=indexing
            tunnel: w416 -> [w432] mode=indexing
            shift-right: [w430] -> w410
            shift-left: w411 -> [w431]
            n172 = property class="Ctl"(reference=w432, error in=w431, "Value"=w434, "Caption.Text"=w433) -> (error out=w430:errorcluster)  [unwired: 1 out]
          }
        }
        frame "6-Dbl Cluster" {
          w469 = refnum<vi> refnum  # 簇
          w464 = TRUE  # Visible
          w465 = T5[] [enum."Escape Key Cancel", enum."Cancel Button", enum."Accept Button", enum."Enter Key Accept", enum."Mouse Outside Cancel"] items=["Nothing", "Enter Key Accept", "Escape Key Cancel", "Mouse Outside Accept", "Mouse Outside Cancel", "Mouse Move Accept", "Mouse Move Cancel", "Mouse Leave Cancel", "Value Change Accept", "Lose Focus Cancel", "Cancel Button", "Accept Button", "Shift Ctrl Key Down"]  # Events to Register
          # "If no caption, or if blank\nDefault is a Rect"
          n173 = Array Size(array=w458) -> (size(s)=w459:i32)
          n174 = call "POP_Position Cluster.vi"("error in (no error)"=w450, "Mouse Coords"=w463, "Ctl Refnum"=w461) -> ("error out"=w453:errorcluster, "Cluster Pos"=w462:cluster{"x":i32, "y":i32})  [unwired: 6 in, 1 out]
          n175 = Variant To Data(error in=w450, type=T8 {"a0"=0.0, "a1"=0.0, "a2"=0.0, "a3"=0.0, "a4"=0.0, "a5"=0.0} ("rect"), Variant=w460) -> (data=w455:T8, error out=w452:errorcluster)
          n176 = case shown="0" w459 {
            tunnel: w458 -> [_ w478 w482 w487 w488]
            tunnel: [string[] ["Left", "Top", "Right", "Bottom"] w477 w481 w486 w488] -> w457
            frame 0 {
            }
            frame 1 {
              n177 = Index Array(array=w478) -> (element=w476:string)  [unwired: 1 in]
              n178 = Build Array(w476, w476, w476, w476) -> (w477:string[])
            }
            frame 2 {
              n179 = Index Array(array=w482) -> (element #1=w480:string, element #2=w479:string)  [unwired: 2 in]
              n180 = Build Array(w480, w479, w479, w479) -> (w481:string[])
            }
            frame 3 {
              n181 = Index Array(array=w487) -> (element #1=w485:string, element #2=w484:string, element #3=w483:string)  [unwired: 3 in]
              n182 = Build Array(w485, w484, w483, w483) -> (w486:string[])
            }
            frame 4, Default {
            }
          }
          n183 = To More Specific Class(target class=w469, reference=w461, error in=w453) -> (specific class reference=w468:refnum<vi>, error out=w467:errorcluster)
          n184 = Cluster To Array(cluster=w455) -> (array=w454:dbl[])
          n185 = property class="Clust"(reference=w468, error in=w467, "Visible"=w464) -> (error out=w466:errorcluster, "Controls[]"=w456:refnum<vi>[])  [unwired: 1 out]
          n186 = for "Value will be shortest - 4 elements" {
            tunnel: w454 -> [w474] mode=indexing
            tunnel: w457 -> [w473] mode=indexing
            tunnel: w456 -> [w472] mode=indexing
            shift-right: [w470] -> w451
            shift-left: w452 -> [w471]
            n187 = property class="Ctl"(reference=w472, error in=w471, "Value"=w474, "Caption.Text"=w473) -> (error out=w470:errorcluster)  [unwired: 1 out]
          }
        }
      }
      n188 = Subtract(x=w29, y=w28) -> (x-y=w27:cluster{i32, i32})
      n189 = property class="Clust"(reference=w31, error in=w21, "Position"=w27, "Visible"=w11) -> (error out=w20:errorcluster)  [unwired: 1 out]
      n190 = Bundle By Name(cluster=w34, "Control"=w25, "Events"=w26) -> (w24:T4)
      n191 = Merge Errors(w20, w19, w18) -> (w17:errorcluster)
    }
    frame Error {
      w489 = T4 {"Control"=refnum, "Events"=[]}  # event data
    }
  }
  "event data" <- w4
  "error out" <- w2
